vi "HXG2saveTimer.vi"(7 "SaveTimerFGV":T1, 8 "error in (no error)":errorcluster, 10 "Interval(s)":dbl, 11 "Duration(min)":dbl) -> (0 "error out":errorcluster, 1 "Dur Done?":bool, 2 "IntDone?":bool, 3 "Int Elapsed(s)":dbl, 5 "Dur Elapsed":dbl)   [LabVIEW 2012]
uses:
  HXG2saveTimer.ctl
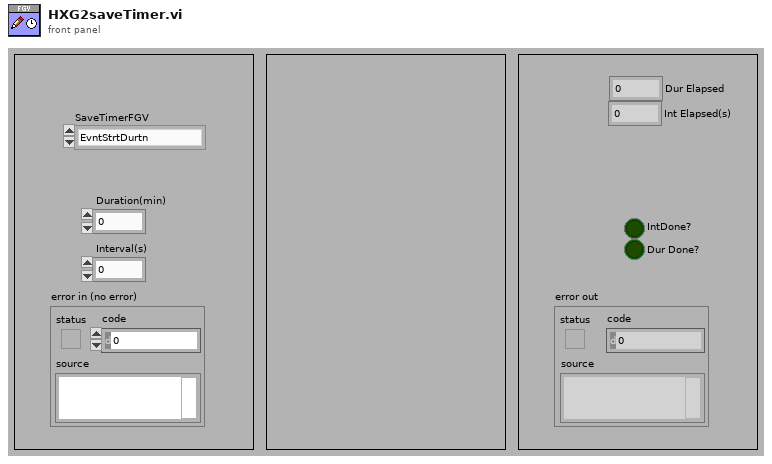
[diagram p1: front panel]
types:
  T1 = typedef "HXG2saveTimer.ctl" = enum16{"EvntStrtDurtn", "EvntStrtInterv", "Stop", "Check", "RegStrtInterv", "Add10Durtn", "Take10Durtn"}
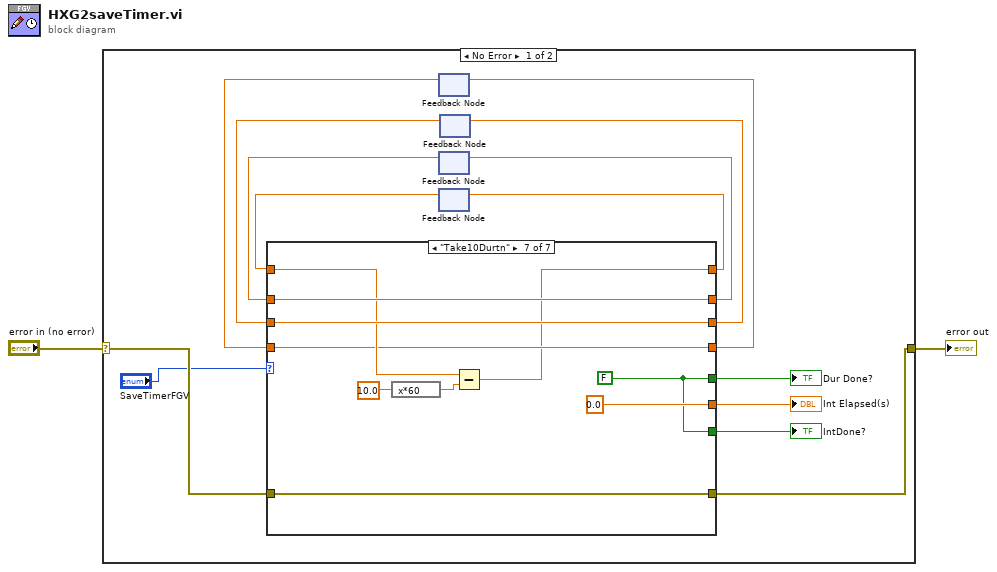
[diagram p0: block diagram]
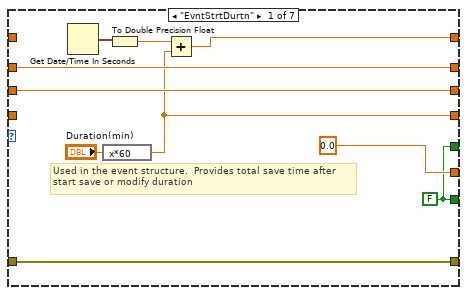
[diagram p2: hidden frame]
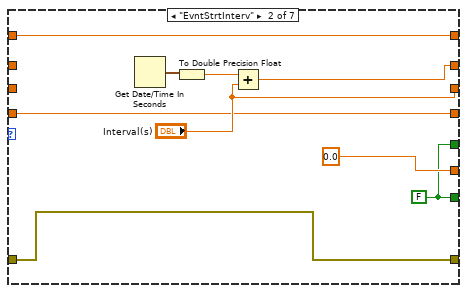
[diagram p3: hidden frame]
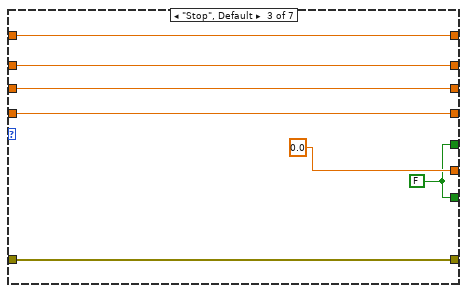
[diagram p4: hidden frame]
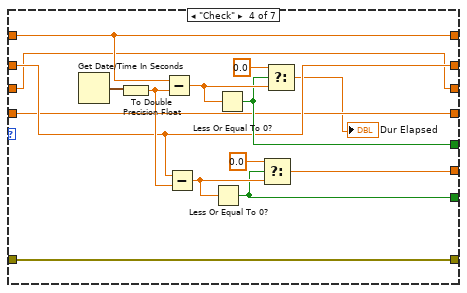
[diagram p5: hidden frame]
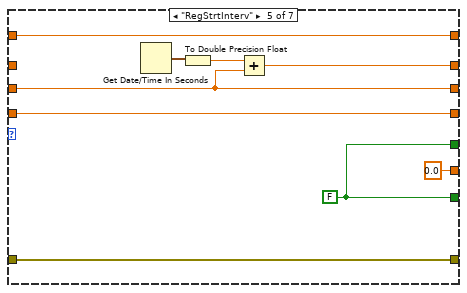
[diagram p6: hidden frame]
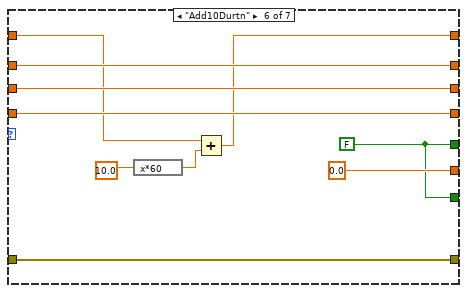
[diagram p7: hidden frame]
diagram:
  n1 = case shown="No Error" "error in (no error)" {
    selector: "error in (no error)" -> [w14 w87]
    tunnel: [w13 w87] -> w1
    frame No Error {
      n2 = feedback #1() -> (w3:dbl)  [unwired: 1 in]
      n3 = feedback #2() -> (w8:dbl)  [unwired: 1 in]
      n4 = feedback #3() -> (w15:dbl)  [unwired: 1 in]
      n5 = feedback #4() -> (w5:dbl)  [unwired: 1 in]
      n6 = case shown="\"Take10Durtn\"" "SaveTimerFGV" {
        tunnel: [w23 w30 w42 w55 w66 w67 w77] -> w16
        tunnel: w15 -> [_ w30 w42 w55 w66 w68 w79]
        tunnel: w14 -> [w26 w35 w41 w56 w59 w76 w86]
        tunnel: [w26 w35 w41 w56 w59 w76 w86] -> w13
        tunnel: [0.0 0.0 0.0 w47 0.0 ("t") 0.0 ("t") 0.0 ("t")] -> w11
        tunnel: [w20 w29 w38 w46 w61 w70 w80] -> w10
        tunnel: [w22 w31 w40 w48 w62 w75 w85] -> w9
        tunnel: w8 -> [w22 _ w40 w48 _ w75 w85]
        tunnel: [w20 w29 w38 w49 w61 w70 w80] -> w7
        tunnel: [w19 "Interval(s)" w37 w45 w63 w74 w84] -> w6
        tunnel: w5 -> [w19 _ w37 w45 w63 w74 w84]
        tunnel: [w17 w27 w36 w44 w60 w69 w78] -> w4
        tunnel: w3 -> [_ w27 w36 w44 w60 w69 w78]
        frame "EvntStrtDurtn" {
          w20 = FALSE
          # "Used in the event structure.  Provides total save time after\nstart save or modify duration"
          n7 = Get Date/Time In Seconds() -> (seconds since 1Jan1904=w25:timestamp)
          n8 = expression code="x*60"("Duration(min)") -> (w17:dbl)
          n9 = To Double Precision Float(number=w25) -> (double precision float=w24:dbl)
          n10 = Add(x=w24, y=w17) -> (x+y=w23:dbl)
        }
        frame "EvntStrtInterv" {
          w29 = FALSE
          n11 = Get Date/Time In Seconds() -> (seconds since 1Jan1904=w34:timestamp)
          n12 = To Double Precision Float(number=w34) -> (double precision float=w33:dbl)
          n13 = Add(x=w33, y="Interval(s)") -> (x+y=w31:dbl)
        }
        frame "Stop", Default {
          w38 = FALSE
        }
        frame "Check" {
          n14 = Get Date/Time In Seconds() -> (seconds since 1Jan1904=w57:timestamp)
          n15 = To Double Precision Float(number=w57) -> (double precision float=w50:dbl)
          n16 = Subtract(x=w55, y=w50) -> (x-y=w54:dbl)
          n17 = Subtract(x=w48, y=w50) -> (x-y=w51:dbl)
          n18 = Less Or Equal To 0?(x=w51) -> (x <= 0?=w46:bool)
          n19 = Less Or Equal To 0?(x=w54) -> (x <= 0?=w49:bool)
          n20 = Select(t=0.0, s=w46, f=w51) -> (s? t:f=w47:dbl)
          n21 = Select(t=0.0, s=w49, f=w54) -> (s? t:f=→"Dur Elapsed":dbl)
        }
        frame "RegStrtInterv" {
          w61 = FALSE
          n22 = Get Date/Time In Seconds() -> (seconds since 1Jan1904=w65:timestamp)
          n23 = To Double Precision Float(number=w65) -> (double precision float=w64:dbl)
          n24 = Add(x=w64, y=w63) -> (x+y=w62:dbl)
        }
        frame "Add10Durtn" {
          w70 = FALSE
          n25 = expression code="x*60"(10.0 ("y")) -> (w71:dbl)
          n26 = Add(x=w68, y=w71) -> (x+y=w67:dbl)
        }
        frame "Take10Durtn" {
          w80 = FALSE
          n27 = expression code="x*60"(10.0 ("y")) -> (w81:dbl)
          n28 = Subtract(x=w79, y=w81) -> (x-y=w77:dbl)
        }
      }
      "Int Elapsed(s)" <- w11
      "IntDone?" <- w10
      "Dur Done?" <- w7
      n29 = feedback-in #1(w4) -> ()
      n30 = feedback-in #2(w9) -> ()
      n31 = feedback-in #3(w16) -> ()
      n32 = feedback-in #4(w6) -> ()
    }
    frame Error {
    }
  }
  "error out" <- w1
